vi "Campus Weather Monitor.vi"() -> ()   [LabVIEW 2011]
uses:
  <vilib>/Analysis/NI_AALBase.lvlib
panel:
  out "Forecast Text":u16(ring) items=["Sunny", "Partially Cloudy", "Scattered Showers", "Cloudy", "Thunderstorm", "Rain"]
  out "Forecast":u16(ring)
  out "Wind Chill Number":dbl format="%#.0p°F"
  out "Wind Chill":dbl(slide)=46.93877551020408 scale=0.0..100.0 scale format="%#_g°F"
  out "Air Temp Number":dbl format="%#.0p°F"
  out "Air Temp":dbl(slide)=46.93877551020408 scale=0.0..100.0 scale format="%#_g°F"
  out "Wind Speed Number":dbl format="%#.0p mph"
  out "Wind Speed":dbl(knob) scale=0.0..20.0
  # "Campus Weather Monitor"
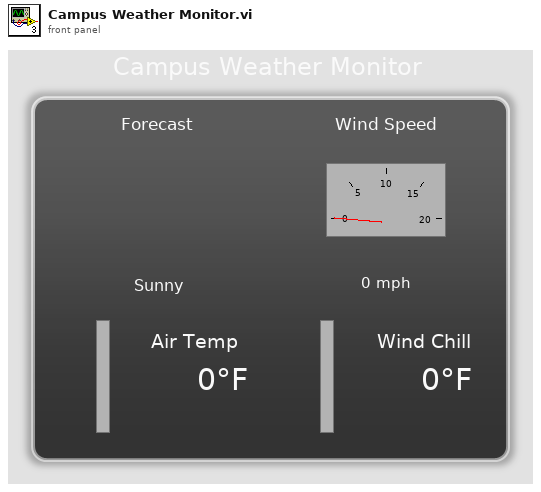
[diagram p1: front panel]
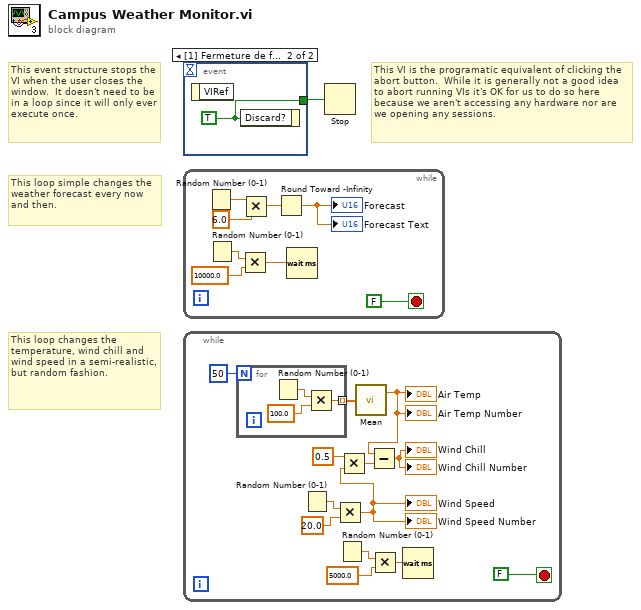
[diagram p0: block diagram]
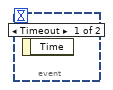
[diagram p2: hidden frame]
diagram:
  # "This loop changes the temperature, wind chill and wind speed in a semi-realistic, but random fashion."
  # "This loop simple changes the weather forecast every now and then."
  # "This VI is the programatic equivalent of clicking the abort button.  While it is generally not a good idea to abort running VIs it's OK for us to do so here because we aren't accessing any hardware nor are we opening any sessions."
  # "This event structure stops the VI when the user closes the window.  It doesn't need to be in a loop since it will only ever execute once."
  n1 = event shown="[1] Fermeture de face-avant ?" {
    selector: _ -> [_ _]
    dyn-events: _ -> [_ _]
    timeout: _ -> [_ _]
    tunnel: [_ w2] -> w1
    event Timeout {
      n2 = event-data() -> ()  [unwired: 1 in, 1 out]
    }
    event Panel Close? {
      w2 = TRUE ("Discard?")
      n3 = event-data() -> ()  [unwired: 1 in, 1 out]
      n4 = event-data("Discard?"=w2) -> ()  [unwired: 1 in, 1 out]
    }
  }
  n5 = while {
    stop <- FALSE stop-if-true
    n6 = Random Number (0-1)() -> (number: 0 to 1=w10:dbl)
    n7 = Random Number (0-1)() -> (number: 0 to 1=w5:dbl)
    n8 = Multiply(x=w5, y=10000.0) -> (x*y=w4:dbl)
    n9 = Multiply(x=w10, y=6.0) -> (x*y=w8:dbl)
    n10 = Round Toward -Infinity(1:w8) -> (0:→"Forecast" →"Forecast Text":dbl)
    n11 = Wait (ms)(milliseconds to wait=w4) -> ()  [unwired: 1 out]
  }
  n12 = while {
    stop <- FALSE stop-if-true
    n13 = for {
      N: 50 -> [_]
      tunnel: [w24] -> w19 mode=indexing
      n14 = Random Number (0-1)() -> (number: 0 to 1=w25:dbl)
      n15 = Multiply(x=w25, y=100.0) -> (x*y=w24:dbl)
    }
    n16 = Random Number (0-1)() -> (number: 0 to 1=w22:dbl)
    n17 = Multiply(x=w22, y=20.0) -> (x*y=w15:dbl)
    "Wind Speed" <- w15
    "Wind Speed Number" <- w15
    n18 = Random Number (0-1)() -> (number: 0 to 1=w12:dbl)
    n19 = Multiply(x=0.5 ("y"), y=w15) -> (x*y=w14:dbl)
    n20 = call <vilib>:"Mean.vi"("X"=w19) -> ("mean"=w17:dbl)  [unwired: 1 out]
    "Air Temp" <- w17
    "Air Temp Number" <- w17
    n21 = Subtract(x=w17, y=w14) -> (x-y=→"Wind Chill Number" →"Wind Chill":dbl)
    n22 = Multiply(x=w12, y=5000.0) -> (x*y=w13:dbl)
    n23 = Wait (ms)(milliseconds to wait=w13) -> ()  [unwired: 1 out]
  }
  n24 = Stop(stop? (T)=w1) -> ()
